vi "ADC_config_fastsweep.vi"(0 "Inst_parameter":T1, 1 "Fast sequence size":u32, 2 "fast sequence divider":u32, 3 "Ramp?":bool=TRUE) -> (5 "Inst_parameter out":T1)   [LabVIEW 2013]
uses:
  <vilib>/DAQmx/create/channels.llb/DAQmx Create Channel (AI-Voltage-Basic).vi
  <vilib>/DAQmx/configure/timing.llb/DAQmx Timing (Sample Clock).vi
  <vilib>/DAQmx/create/channels.llb/DAQmx Create Channel (CO-Pulse Generation-Frequency).vi
  <vilib>/DAQmx/configure/timing.llb/DAQmx Timing (Implicit).vi
  <vilib>/DAQmx/configure/trigger.llb/DAQmx Start Trigger (Digital Edge).vi
  <resource>/objmgr/daqmx.rc
panel:
  out "error out":errorcluster
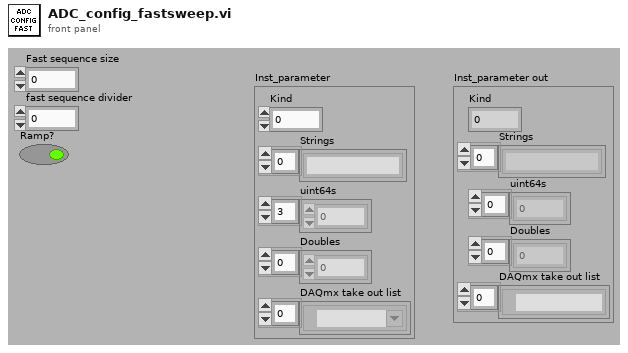
[diagram p1: front panel]
types:
  T1 = cluster{"Kind":u16, "Strings":string[], "uint64s":u64[], "Doubles":dbl[], "DAQmx take out list":refnum<k21>[]}
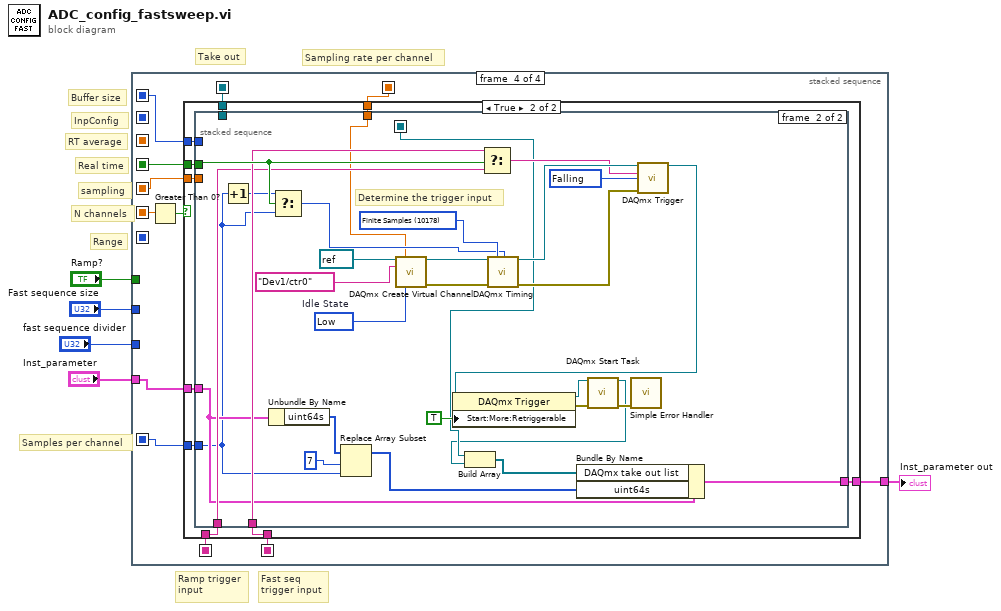
[diagram p0: block diagram]
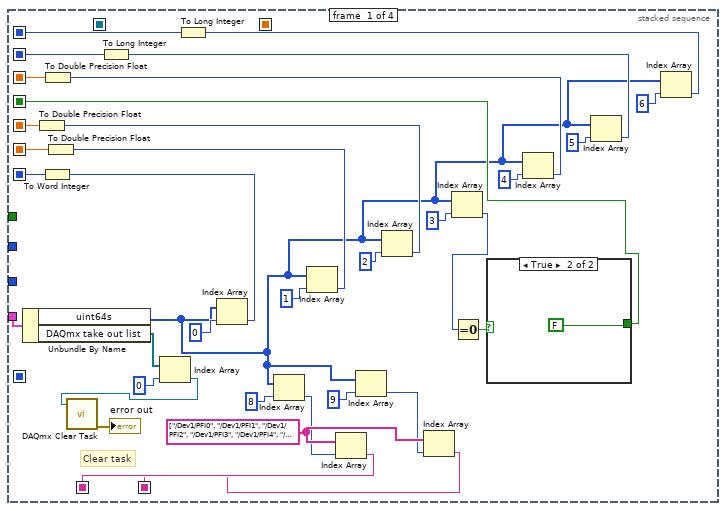
[diagram p2: hidden frame]
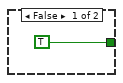
[diagram p3: hidden frame]
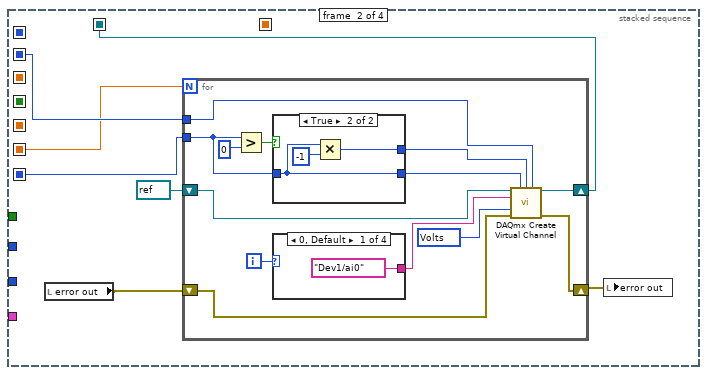
[diagram p4: hidden frame]
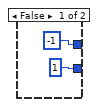
[diagram p5: hidden frame]
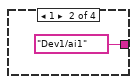
[diagram p6: hidden frame]
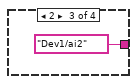
[diagram p7: hidden frame]
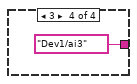
[diagram p8: hidden frame]
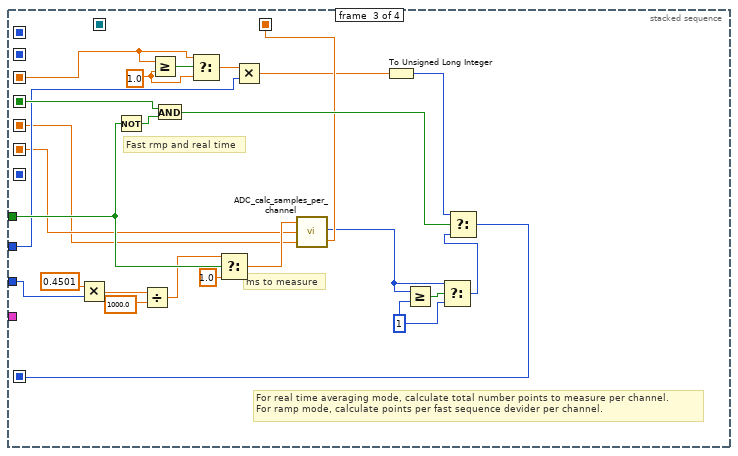
[diagram p9: hidden frame]
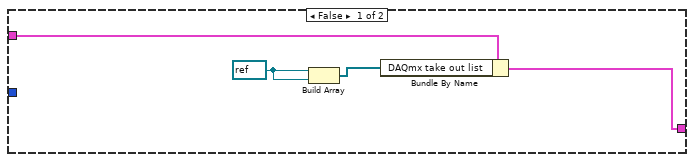
[diagram p10: hidden frame]
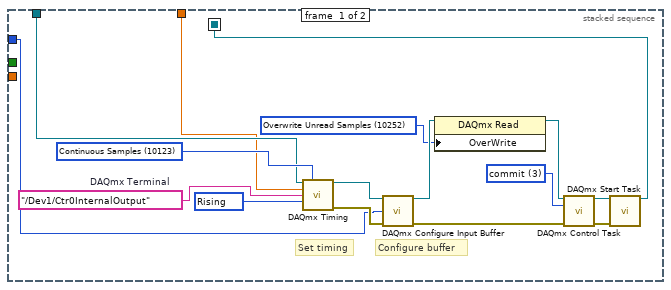
[diagram p11: hidden frame]
diagram:
  # "Fast seq \ntrigger input"
  # "Ramp trigger\ninput"
  # "Take out"
  # "Sampling rate per channel"
  # "Samples per channel"
  # "Buffer size"
  # "InpConfig"
  # "RT average"
  # "Real time"
  # "sampling"
  # "N channels"
  # "Range"
  n1 = stacked-sequence {
    seq-local: [w25 _ _ _] -> [_ _ _ w105]
    seq-local: [w20 _ _ _] -> [_ w48 _ _]
    seq-local: [w23 _ _ _] -> [_ _ w72 _]
    seq-local: [w17 _ _ _] -> [_ _ w97 w104]
    seq-local: [w22 _ _ _] -> [_ _ w81 w98]
    seq-local: [w24 _ _ _] -> [_ w44 w82 w109]
    seq-local: [w21 _ _ _] -> [_ w47 _ _]
    seq-local: [_ _ w75 _] -> [_ _ _ w103]
    seq-local: [_ _ w84 _] -> [_ _ _ w107]
    seq-local: [_ w43 _ _] -> [_ _ _ w106]
    seq-local: [w7 _ _ _] -> [_ _ _ w101]
    seq-local: [w6 _ _ _] -> [_ _ _ w102]
    tunnel: "Inst_parameter" -> [w39 _ _ w100]
    tunnel: "Fast sequence size" -> [_ _ w85 _]
    tunnel: "fast sequence divider" -> [_ _ w91 _]
    tunnel: "Ramp?" -> [_ _ w95 _]
    tunnel: [_ _ _ w99] -> w1
    frame #0 {
      w10 = tag[] ["/Dev1/PFI0", "/Dev1/PFI1", "/Dev1/PFI2", "/Dev1/PFI3", "/Dev1/PFI4", "/Dev1/PFI5", "/Dev1/PFI6", "/Dev1/PFI7", "/Dev1/PFI8", "/Dev1/PFI9", "/Dev1/PFI10", "/Dev1/PFI11", "/Dev1/PFI12"]
      # "Clear task"
      n2 = Unbundle By Name(w39) -> ("uint64s"=w13:u64[], "DAQmx take out list"=w15:refnum<k21>[])
      n3 = Index Array(array=w15, index=0) -> (element=w14:refnum<k21>)
      n4 = call <vilib>:"DAQmx Clear Task.vi"("task in"=w14) -> ("error out"=→"error out":errorcluster)  [unwired: 14 in]
      n5 = Index Array(array=w13, index=0) -> (element=w26:u64)
      n6 = To Word Integer(number=w26) -> (16bit integer=w21:i16)
      n7 = Index Array(array=w13, index=8) -> (element=w9:u64)
      n8 = Index Array(array=w13, index=1) -> (element=w27:u64)
      n9 = To Double Precision Float(number=w27) -> (double precision float=w24:dbl)
      n10 = Index Array(array=w10, index=w9) -> (element=w7:tag)
      n11 = Index Array(array=w13, index=9) -> (element=w8:u64)
      n12 = Index Array(array=w13, index=2) -> (element=w28:u64)
      n13 = To Double Precision Float(number=w28) -> (double precision float=w22:dbl)
      n14 = Index Array(array=w10, index=w8) -> (element=w6:tag)
      n15 = Index Array(array=w13, index=3) -> (element=w18:u64)
      n16 = Equal To 0?(x=w18) -> (x = 0?=w19:bool)
      n17 = case shown="True" w19 {
        tunnel: [TRUE FALSE] -> w17
        frame False {
        }
        frame True {
        }
      }
      n18 = Index Array(array=w13, index=4) -> (element=w29:u64)
      n19 = To Double Precision Float(number=w29) -> (double precision float=w23:dbl)
      n20 = Index Array(array=w13, index=5) -> (element=w30:u64)
      n21 = To Long Integer(number=w30) -> (32bit integer=w20:i32)
      n22 = Index Array(array=w13, index=6) -> (element=w31:u64)
      n23 = To Long Integer(number=w31) -> (32bit integer=w25:i32)
    }
    frame #1 {
      n24 = local read "error out"() -> (w46:errorcluster)
      n25 = for {
        N: w44 -> [_]
        shift-right: [w62] -> w43
        shift-left: refnum<k21> refnum ("task out") -> [w61]
        shift-right: [w58] -> w45
        shift-left: w46 -> [w57]
        tunnel: w47 -> [w54]
        tunnel: w48 -> [w50]
        i -> [w51]
        w59 = 10348 items=["Volts"=10348, "From Custom Scale"=10065] ("units")
        n26 = Greater?(x=w54, y=i16 0) -> (0:w55:bool)
        n27 = case shown="True" w55 {
          tunnel: w54 -> [_ w65]
          tunnel: [i16 -1 w66] -> w56
          tunnel: [i16 1 ("Range") w65] -> w52
          frame False {
          }
          frame True {
            n28 = Multiply(x=w65, y=i16 -1) -> (x*y=w66:i16)
          }
        }
        n29 = case shown="0, Default" w51 {
          tunnel: [tag "Dev1/ai0" ("physical channels") tag "Dev1/ai1" ("physical channels") tag "Dev1/ai2" ("physical channels") tag "Dev1/ai3" ("physical channels")] -> w60
          frame 0, Default {
          }
          frame 1 {
          }
          frame 2 {
          }
          frame 3 {
          }
        }
        n30 = call-poly <vilib>:"DAQmx Create Virtual Channel.vi"("task in"=w61, "maximum value"=w52, "minimum value"=w56, "input terminal configuration"=w50, "physical channels"=w60, "units"=w59, "error in"=w57) -> ("task out"=w62:refnum<k21>, "error out"=w58:errorcluster)  [unwired: 2 in, 5 out]
      }
      n31 = local write "error out"(w45) -> ()
    }
    frame #2 {
      w79 = 1
      w74 = 1.0 ("t")
      # "For real time averaging mode, calculate total number points to measure per channel.\nFor ramp mode, calculate points per fast sequence devider per channel."
      # "ms to measure"
      # "Fast rmp and real time"
      n32 = Multiply(x=0.4501, y=w91) -> (x*y=w93:dbl)
      n33 = Not(x=w95) -> (.not. x?=w96:bool)
      n34 = Divide(x=w93, y=1000.0) -> (x/y=w90:dbl)
      n35 = Greater Or Equal?(x=w72, y=w74) -> (x >= y?=w73:bool)
      n36 = And(x=w97, y=w96) -> (x .and. y?=w87:bool)
      n37 = Select(t=w72, s=w73, f=w74) -> (s? t:f=w86:dbl)
      n38 = Select(t=w90, s=w95, f=1.0) -> (s? t:f=w83:dbl)
      n39 = Multiply(x=w86, y=w85) -> (x*y=w77:dbl)
      n40 = call "ADC_calc_samples_per_channel.vi"("Samplingrate"=w81, "Nchannel"=w82, "time per point (ms)"=w83) -> ("effective samplingrate"=w84:dbl, "samples to read"=w78:u32)
      n41 = To Unsigned Long Integer(number=w77) -> (unsigned 32bit integer=w76:u32)
      n42 = Greater Or Equal?(x=w78, y=w79) -> (x >= y?=w80:bool)
      n43 = Select(t=w78, s=w80, f=w79) -> (s? t:f=w88:u32)
      n44 = Select(t=w76, s=w87, f=w88) -> (s? t:f=w75:u32)
    }
    frame #3 {
      n45 = Greater Than 0?(x=w109) -> (x > 0?=w108:bool)
      n46 = case shown="True" w108 {
        tunnel: w107 -> [_ w123]
        tunnel: w106 -> [_ w122]
        tunnel: w105 -> [_ w121]
        tunnel: w104 -> [_ w120]
        tunnel: w103 -> [_ w119]
        tunnel: w102 -> [_ w118]
        tunnel: w101 -> [_ w117]
        tunnel: w100 -> [w113 w116]
        tunnel: [w110 w115] -> w99
        tunnel: w98 -> [_ w114]
        frame False {
          w112 = refnum<k21> refnum ("task out")
          n47 = Build Array(w112, w112) -> (w111:refnum<k21>[])
          n48 = Bundle By Name(cluster=w113, "DAQmx take out list"=w111) -> (w110:T1)
        }
        frame True {
          n49 = stacked-sequence {
            seq-local: [w125 _] -> [_ w152]
            tunnel: w123 -> [w124 w140]
            tunnel: w122 -> [w127 _]
            tunnel: w121 -> [w126 _]
            tunnel: w120 -> [_ w154]
            tunnel: w119 -> [_ w142]
            tunnel: w118 -> [_ w150]
            tunnel: w117 -> [_ w149]
            tunnel: w116 -> [_ w148]
            tunnel: [_ w143] -> w115
            tunnel: w114 -> [_ _]
            frame #0 {
              w128 = 10252 items=["Overwrite Unread Samples"=10252, "Do Not Overwrite Unread Samples"=10159] ("OverWrite")
              w130 = 3 items=["verify"=2, "reserve"=4, "commit"=3, "unreserve"=5, "abort"=6] ("action")
              w137 = tag "/Dev1/Ctr0InternalOutput"  # DAQmx Terminal
              w138 = 10280 items=["Rising"=10280, "Falling"=10171] ("active edge")
              w139 = 10123 items=["Finite Samples"=10178, "Continuous Samples"=10123, "Hardware Timed Single Point"=12522] ("sample mode")
              # "Set timing"
              # "Configure buffer"
              n50 = call-poly <vilib>:"DAQmx Timing.vi"("task/channels in"=w127, "sample mode"=w139, "rate"=w124, "source"=w137, "active edge"=w138) -> ("task out"=w136:refnum<k21>, "error out"=w135:errorcluster)  [unwired: 9 in]
              n51 = call <vilib>:"DAQmx Configure Input Buffer.vi"("task/channels in"=w136, "buffer size (in samples per channel)"=w126, "error in"=w135) -> ("task out"=w134:refnum<k21>, "error out"=w132:errorcluster)  [unwired: 11 out]
              n52 = property class="DAQmx Read"(reference=w134, "OverWrite"=w128) -> (reference out=w129:refnum<k21>)  [unwired: 1 in, 1 out]
              n53 = call <vilib>:"DAQmx Control Task.vi"("task/channels in"=w129, "action"=w130, "error in"=w132) -> ("task out"=w133:refnum<k21>, "error out"=w131:errorcluster)  [unwired: 11 in]
              n54 = call <vilib>:"DAQmx Start Task.vi"("task/channels in"=w133, "error in"=w131) -> ("task out"=w125:refnum<k21>)  [unwired: 12 in, 1 out]
            }
            frame #1 {
              w163 = 10171 items=["Rising"=10280, "Falling"=10171] ("Trigger Edge")
              w166 = 10214 items=["High"=10192, "Low"=10214]  # Idle State
              w167 = 10178 items=["Finite Samples"=10178, "Continuous Samples"=10123] ("sample mode")
              # "Determine the trigger input"
              n55 = Increment(x=w142) -> (x+1=w141:u32)
              n56 = Unbundle By Name(w148) -> ("uint64s"=w146:u64[])
              n57 = Select(t=w141, s=w154, f=w142) -> (s? t:f=w153:u32)
              n58 = Replace Array Subset(array=w146, new element=w142, index=7) -> (w144:u64[])
              n59 = call-poly <vilib>:"DAQmx Create Virtual Channel.vi"("task in"=refnum<k21> refnum, "frequency"=w140, "counter"=tag "Dev1/ctr0", "idle state"=w166) -> ("task out"=w168:refnum<k21>, "error out"=w169:errorcluster)  [unwired: 5 in, 5 out]
              n60 = Select(t=w150, s=w154, f=w149) -> (s? t:f=w161:tag)
              n61 = call-poly <vilib>:"DAQmx Timing.vi"("task/channels in"=w168, "sample mode"=w167, "samples per channel"=w153, "error in"=w169) -> ("task out"=w165:refnum<k21>, "error out"=w164:errorcluster)  [unwired: 2 in, 8 out]
              n62 = call-poly <vilib>:"DAQmx Trigger.vi"("task/channels in"=w165, "source"=w161, "edge"=w163, "error in"=w164) -> ("task out"=w156:refnum<k21>)  [unwired: 11 out]
              n63 = property class="DAQmx Trigger"(reference=w156, "Start:More:Retriggerable"=TRUE) -> (reference out=w155:refnum<k21>, error out=w158:errorcluster)  [unwired: 1 in]
              n64 = call <vilib>:"DAQmx Start Task.vi"("task/channels in"=w155, "error in"=w158) -> ("task out"=w151:refnum<k21>, "error out"=w157:errorcluster)  [unwired: 12 out]
              n65 = Build Array(w152, w151) -> (w147:refnum<k21>[])
              n66 = Bundle By Name(cluster=w148, "DAQmx take out list"=w147, "uint64s"=w144) -> (w143:T1)
              n67 = call <vilib>:"Simple Error Handler.vi"("error in (no error)"=w157) -> ()  [unwired: 4 in, 5 out]
            }
          }
        }
      }
    }
  }
  "Inst_parameter out" <- w1
